vi "LaserLineDetection_Intensity_detect.vi"(0 "Source In":T1=refnum, 1 "F = I_max\nT = Gauss":bool, 2 "F = Gauss S\nT = Gauss ES":bool, 9 "index":i32, 11 "Error In":errorcluster, 12 "Laser Detected Old":bool) -> (3 "appended array":cluster{u8[], i32[]}[](array[cluster]), 4 "Source Out":T1, 6 "Distance to Wall (m)":dbl, 8 "delta° (incident angle)":dbl, 10 "Perpendicular Distance to Wall (m)":dbl, 13 "Laser Detected":bool, 14 "Laser Detected Twice":bool, 15 "Error Out":errorcluster)   [LabVIEW 2013]
uses:
  <vilib>/vision/Image Controls.llb/IMAQ Image.ctl
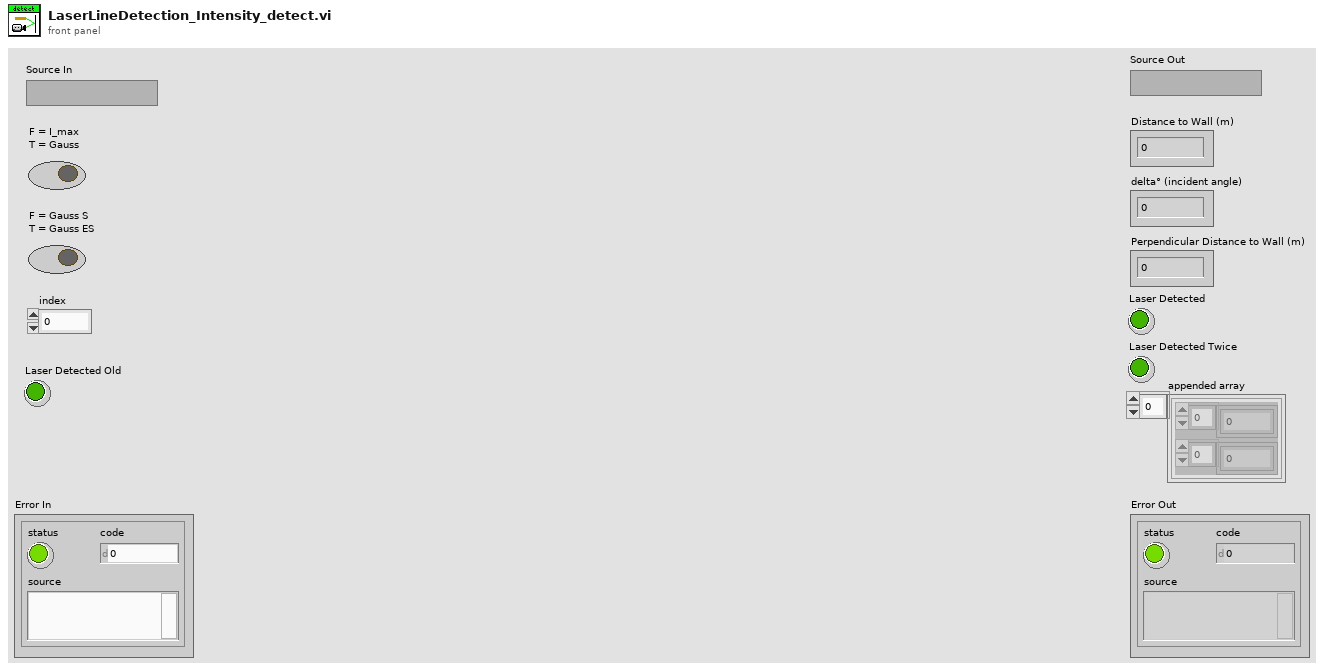
[diagram p1: front panel]
types:
  T1 = typedef "IMAQ Image.ctl" = refnum<image>
  T2 = cluster{"Horizontal Resolution":dbl, "Vertical Resolution":dbl, "alpha° (horizontal)":dbl, "beta° (vertical)":dbl, "distance to Laser (dL)":dbl}
  T3 = cluster{"Left":i32, "Top":i32, "Right":i32, "Bottom":i32}
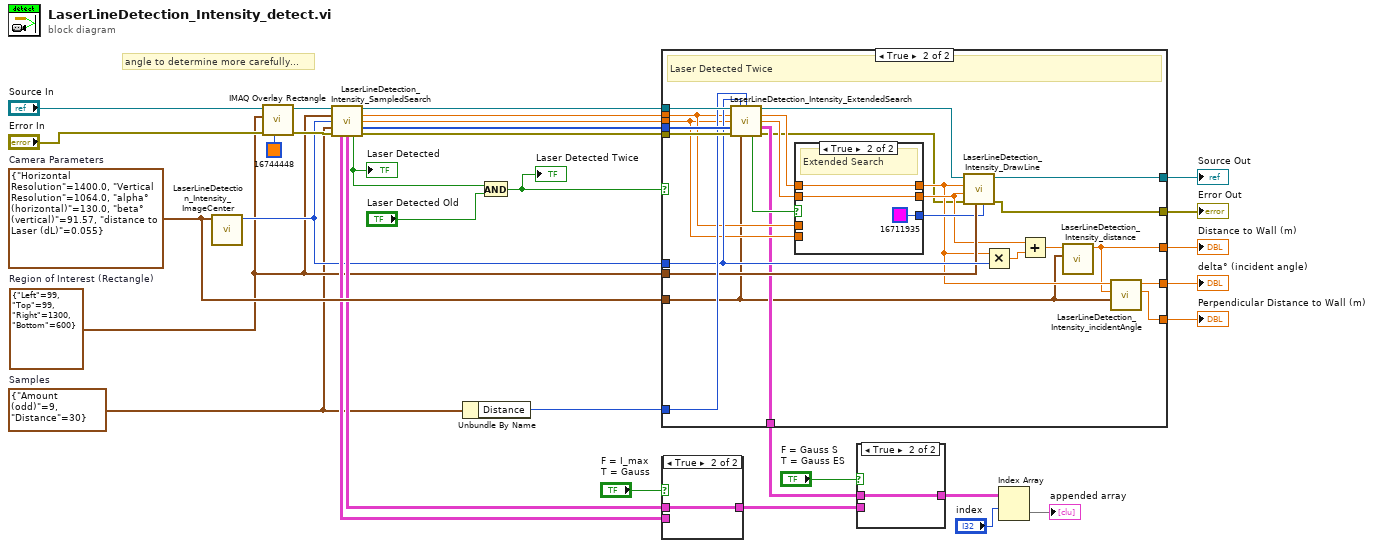
[diagram p0: block diagram]
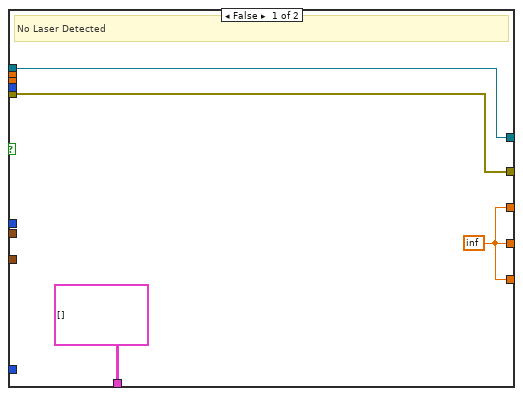
[diagram p4: hidden frame]
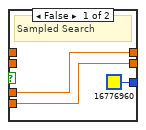
[diagram p5: hidden frame]
diagram:
  w5 = cluster{"Amount (odd)":i32, "Distance":i32} {"Amount (odd)"=9, "Distance"=30}  # Samples
  w27 = T2 {"Horizontal Resolution"=1400.0, "Vertical Resolution"=1064.0, "alpha° (horizontal)"=130.0, "beta° (vertical)"=91.57, "distance to Laser (dL)"=0.055}  # Camera Parameters
  w6 = T3 {"Left"=99, "Top"=99, "Right"=1300, "Bottom"=600}  # Region of Interest (Rectangle)
  # "angle to determine more carefully..."
  n1 = call "LaserLineDetection_Intensity_ImageCenter.vi"("Camera Parameters"=w27) -> ("Image Center (Horizontal)"=w7:i32)  [unwired: 10 in]
  n2 = call "IMAQ Overlay Rectangle"("Color"=u32 16744448, "error in (no error)"="Error In", "Rectangle"=w6, "Image"="Source In") -> ("error out"=w15:errorcluster, "Image Out"=w16:T1)  [unwired: 6 in]
  n3 = call "LaserLineDetection_Intensity_SampledSearch.vi"("Image In"=w16, "Region of Interest (Rectangle)"=w6, "Image Center (Horizontal)"=w7, "Samples"=w5, "error in (no error)"=w15) -> ("Image Out"=w13:T1, "slope SS"=w12:dbl, "intercept SS"=w11:dbl, "INTENSITYarray SS"=w10:u8[], "appended array Imax"=w9:cluster{u8[], i32[]}[][], "appended array Gauss"=w8:cluster{u8[], i32[]}[][], "Sampled Search Accepted"=w3:bool, "error out"=w14:errorcluster)  [unwired: 3 in]
  "Laser Detected" <- w3
  n4 = Unbundle By Name(w5) -> ("Distance"=w19:i32)
  n5 = And(x=w3, y="Laser Detected Old") -> (x .and. y?=w2:bool)
  "Laser Detected Twice" <- w2
  n6 = case shown="True" w2 {
    tunnel: w6 -> [_ w55]
    tunnel: w7 -> [_ w56]
    tunnel: [w36 w47] -> w29
    tunnel: [w35 w48] -> w28
    tunnel: w27 -> [_ w39]
    tunnel: [w33 w41] -> w26
    tunnel: [w33 w43] -> w25
    tunnel: w13 -> [w36 w60]
    tunnel: w14 -> [w35 w59]
    tunnel: w12 -> [_ w52]
    tunnel: w11 -> [_ w51]
    tunnel: w19 -> [_ w57]
    tunnel: w10 -> [_ w58]
    tunnel: [cluster{u8[], i32[]}[][] [] ("appended array") w46] -> w20
    tunnel: [w33 w42] -> w1
    frame False {
      w33 = inf
      # "No Laser Detected"
    }
    frame True {
      # "Laser Detected Twice"
      n7 = call "LaserLineDetection_Intensity_ExtendedSearch.vi"("Image In"=w60, "Image Center (Horizontal)"=w56, "Search Distance"=w57, "slope In"=w52, "intercept In"=w51, "INTENSITYarray"=w58, "error in (no error)"=w59, "Camera Parameters"=w39) -> ("Image Out"=w37:T1, "slope ES"=w50:dbl, "intercept ES"=w49:dbl, "appended array"=w46:cluster{u8[], i32[]}[][], "Extended Search Accepted"=w54:bool, "error out"=w38:errorcluster)  [unwired: 2 in]
      n8 = case shown="True" w54 {
        tunnel: [u32 16776960 ("Color") u32 16711935 ("Color")] -> w53
        tunnel: w52 -> [w63 _]
        tunnel: [w63 w67] -> w44
        tunnel: w51 -> [w62 _]
        tunnel: [w62 w66] -> w45
        tunnel: w50 -> [_ w67]
        tunnel: w49 -> [_ w66]
        frame False {
          # "Sampled Search"
        }
        frame True {
          # "Extended Search"
        }
      }
      n9 = call "LaserLineDetection_Intensity_DrawLine.vi"("Color"=w53, "Region of Interest (Rectangle)"=w55, "error in (no error)"=w38, "intercept"=w45, "slope"=w44, "Refnum in"=w37) -> ("error out"=w48:errorcluster, "Image Out"=w47:T1)  [unwired: 4 in]
      n10 = Multiply(x=w44, y=w56) -> (x*y=w61:dbl)
      n11 = Add(x=w45, y=w61) -> (x+y=w40:dbl)
      n12 = call "LaserLineDetection_Intensity_distance.vi"("Camera Parameters"=w39, "Pixel"=w40) -> ("Distance (D)"=w41:dbl)  [unwired: 9 in]
      n13 = call "LaserLineDetection_Intensity_incidentAngle.vi"("Camera Parameters"=w39, "Distance (D)"=w41, "slope"=w44) -> ("Perpendicular Distance (Dp)"=w42:dbl, "delta° (incident angle)"=w43:dbl)  [unwired: 7 in]
    }
  }
  "Source Out" <- w29
  "Error Out" <- w28
  "Distance to Wall (m)" <- w26
  "delta° (incident angle)" <- w25
  "Perpendicular Distance to Wall (m)" <- w1
  n14 = case shown="True" "F = I_max\nT = Gauss" {
    tunnel: w8 -> [_ w69]
    tunnel: [w68 w69] -> w17
    tunnel: w9 -> [w68 _]
    frame False {
    }
    frame True {
    }
  }
  n15 = case shown="True" "F = Gauss S\nT = Gauss ES" {
    tunnel: w17 -> [w70 _]
    tunnel: [w70 w71] -> w21
    tunnel: w20 -> [_ w71]
    frame False {
    }
    frame True {
    }
  }
  n16 = Index Array(array=w21, index (row)="index") -> (element=→"appended array":cluster{u8[], i32[]}[])  [unwired: 1 in]
